vi "GetMetadataCount.vi"(8 "error in (no error)":errorcluster, 11 "session id in":i32) -> (0 "error out":errorcluster, 2 "MetadataCount":i32, 3 "session id out":i32)   [LabVIEW 2017, in "libonnx_wrapper.lvlib"]
doc: "/**\n * @brief Получить количество метаданных модели\n * \n * ONNX модели могут содержать метаданные: версию, имя автора, описание и т.д.\n * \n * @param sessionId [IN] ID сессии\n * \n * @return int32: Количество пар ключ-значение\n * @return int32: 0 если сессия не найдена или метаданных нет\n */\nint GetMetadataCount(int sessionId);"
uses:
  libonnx_wrapper.lvlib
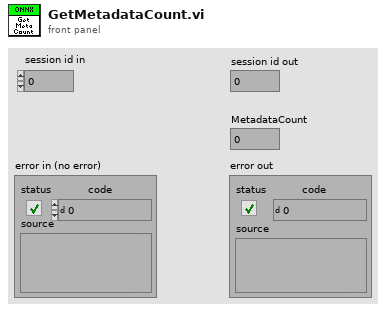
[diagram p1: front panel]
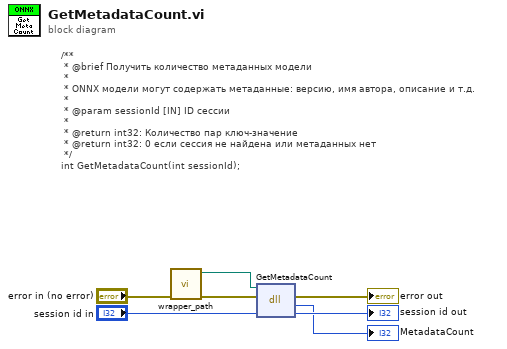
[diagram p0: block diagram]
diagram:
  # "/**\n * @brief Получить количество метаданных модели\n * \n * ONNX модели могут содержать метаданные: версию, имя автора, описание и т.д.\n * \n * @param sessionId [IN] ID сессии\n * \n * @return int32: Количество пар ключ-значение\n * @return int32: 0 если сессия не найдена или метаданных нет\n */\nint GetMetadataCount(int sessionId);"
  n1 = call "wrapper_path.vi"("error in (no error)"="error in (no error)") -> ("error out"=w5:errorcluster, "wrapper path"=w4:path)  [unwired: 9 in]
  n2 = dll-call lib="home/ivan/LabVIEWData/ONNX/Test/libonnx_wrapper/unix64/libonnx_wrapper.so" fn="GetMetadataCount"(path in=w4, error in=w5, "sessionId"="session id in") -> (error out=→"error out":errorcluster, "MetadataCount"=→"MetadataCount":i32, "sessionId"=→"session id out":i32)  [unwired: 1 in, 1 out]
